vi "VALEW_ATC_Verify Concurrent All Valves.vi"(0 "GEA2 Reference In":refnum<k24>, 11 "Error In":errorcluster) -> (4 "GEA2 Reference Out":refnum<k24>, 6 "Pass/fail?":bool, 8 "Report Text":string, 15 "Error Out":errorcluster)   [LabVIEW 2016, in "TL27.lvlib"]
doc: "This test covers the ATC algorithm when doing a concurrent fill with ALL valves. A concurrent fill allows both hot and cold valves to be on at the same time. The valves are operated in parallel. When the cold valve is requested to be on, the fabric softener and spray valves also come on in this test."
uses:
  Projects/TL27.lvlib
  C:/Automation/DLLs/PC Dot Net/GeaCommunication.dll
  Common/LabVIEW GEA2 Toolkit/LabVIEW_GEA2_Toolkit.lvlibp/type defs/Source_Destination.ctl
  Valew Common/type defs/MC_Cycle_Engine_Request_State.ctl
  Common/LabVIEW GEA2 Toolkit/LabVIEW_GEA2_Toolkit.lvlibp/type defs/ERD Write Data In.ctl
  Common/LabVIEW GEA2 Toolkit/LabVIEW_GEA2_Toolkit.lvlibp/type defs/Data Type.ctl
  Common/LabVIEW GEA2 Toolkit/LabVIEW_GEA2_Toolkit.lvlibp/type defs/ERD Read Data In.ctl
  <vilib>/DAQmx/write.llb/DAQmx Write (Analog DBL 1Chan 1Samp).vi
  <vilib>/DAQmx/create/channels.llb/DAQmx Create Channel (AO-Voltage-Basic).vi
  <vilib>/DAQmx/miscellaneous.llb/DAQmx Fill In Error Info.vi
  Common/LabVIEW GEA2 Toolkit/LabVIEW_GEA2_Toolkit.lvlibp
panel:
  out "Calc bath temp after seg gals":dbl
  out "Bath temp after seg gals":dbl
  out "Hot valve time (s) ATC":u16
  out "Cold valve time (s) ATC":u16
  out "Bath temp updated after segment fill?":bool
  out "Valve ON Times (s)":dbl[](array[numeric])
  out "Cold valve pass?":bool
  out "Hot valve pass?":bool
  out "Cold valve time (s) Calc":dbl
  out "Hot valve time (s) Calc":dbl
  in  "Standalone?":bool
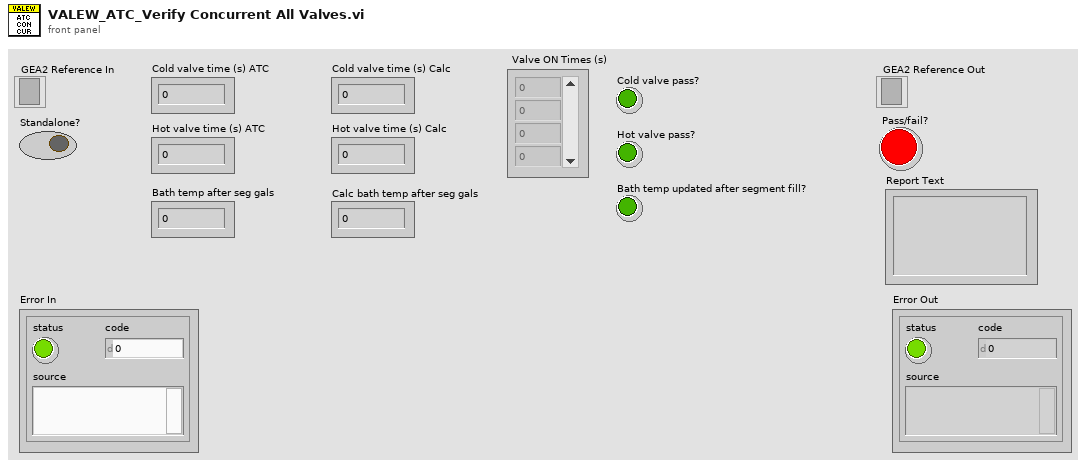
[diagram p1: front panel]
types:
  T1 = typedef "LabVIEW_GEA2_Toolkit.lvlibp/ERD Write Data In.ctl" = cluster{"ERD Number":u16, "Data Type":T2, "Data":string}
  T2 = typedef "LabVIEW_GEA2_Toolkit.lvlibp/Data Type.ctl" = enum16{"string", "boolean", "uint8_t", "uint16_t", "uint32_t", "uint64_t", "int8_t", "int16_t", "int32_t", "int64_t"}
  T3 = typedef "TL27.lvlib/MC_Cycle_Engine_Request_State.ctl" = enum16{"Select", "Start", "Pause", "Resume", "Stop"}
  T4 = typedef "LabVIEW_GEA2_Toolkit.lvlibp/ERD Read Data In.ctl" = cluster{"ERD Number":u16, "Data Type":T2}
  T5 = enum16{"EQ (==)", "NE (!=)", "GT (>)", "LT (<)", "GE (>=)", "LE (<=)", "GTLT(> <)", "GELE (>= <=)", "GELT (>= <)", "GTLE (> <=)", "LTGT (< >)", "LEGE (<= >=)", "LEGT (<= >)", "LTGE (< >=)", "No Comparison"}
  T6 = typedef "LabVIEW_GEA2_Toolkit.lvlibp/Source_Destination.ctl" = cluster{"Source":u8, "Destination":u8}
  T7 = typedef "TL27.lvlib/VALEW_ATC_Data.ctl" = cluster{"Accumulated hot gallons":dbl, "Accumulated cold gallons":dbl, "Current tub gallons":dbl, "Cold inlet temp (F)":dbl, "Hot inlet temp (F)":dbl, "Warm inlet temp (F)":dbl, "Hot valve time (s)":u16, "Cold valve time (s)":u16, "Current bath temp (F)":dbl, "Current water temp (F)":dbl, "Segment gallons":dbl}
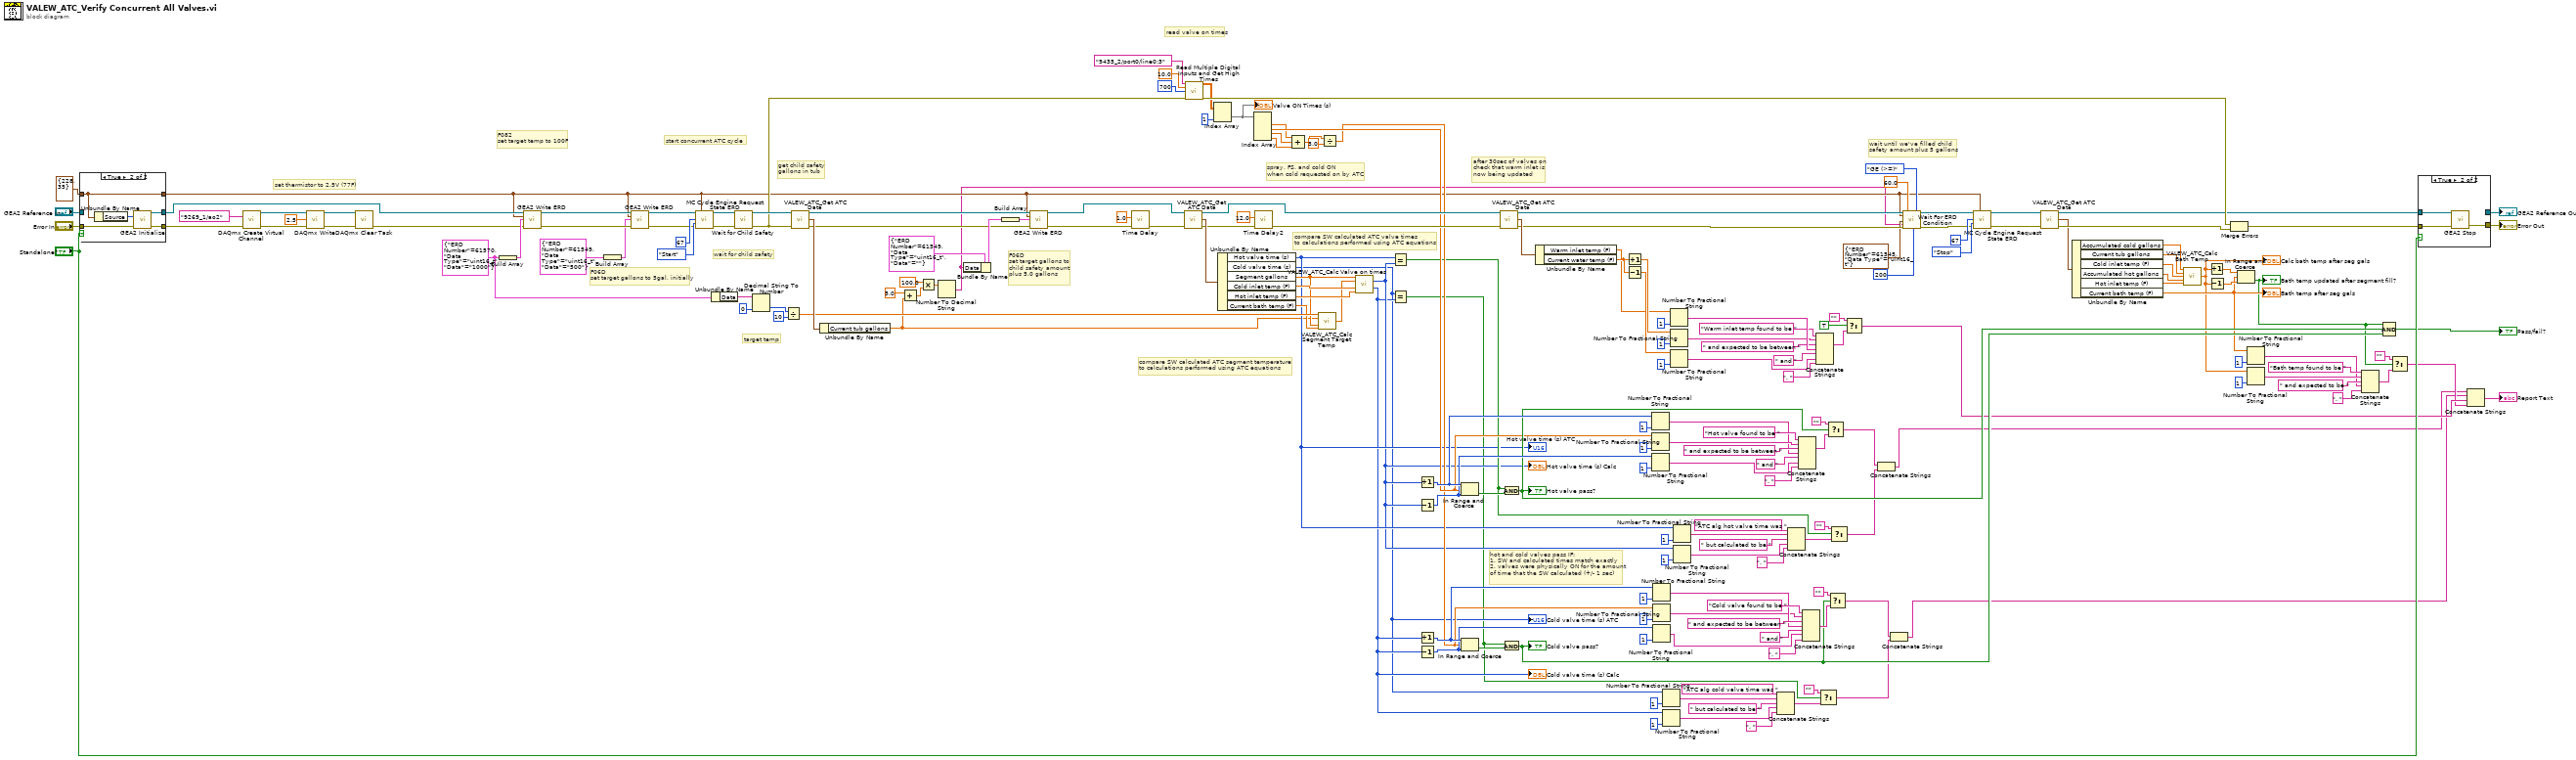
[diagram p0: block diagram]
diagram:
  w184 = T1 {"ERD Number"=61570, "Data Type"=enum."uint16_t", "Data"="1000"} ("ERD Write Data In")
  # "hot and cold valves pass IF:\n1. SW and calculated times match exactly\n2. valves were physically ON for the amount\nof time that the SW calculated (+/- 1 sec)"
  # "compare SW calculated ATC segment temperature\nto calculations performed using ATC equations"
  # "compare SW calculated ATC valve times\nto calculations performed using ATC equations"
  # "F06D\nset target gallons to\nchild safety amount\nplus 5.0 gallons"
  # "spray, FS, and cold ON\nwhen cold requested on by ATC"
  # "F06D\nset target gallons to 5gal, initially"
  # "after 30sec of valves on\ncheck that warm inlet is\nnow being updated"
  # "get child safety\ngallons in tub"
  # "wait until we've filled child \nsafety amount plus 5 gallons"
  # "read valve on times"
  # "target temp"
  # "set thermistor to 2.5V (77F)"
  # "wait for child safety"
  # "start concurrent ATC cycle"
  # "F082\nset target temp to 100F"
  n1 = case shown="True" "Standalone?" {
    tunnel: T6 {"Source"=228, "Destination"=35} ("GEA Inputs") -> [w195 w198]
    tunnel: [w197 w201] -> w48
    tunnel: [w196 w200] -> w138
    tunnel: "Error In" -> [w196 w199]
    tunnel: "GEA2 Reference In" -> [w197 _]
    tunnel: [w195 w198] -> w5
    frame False {
    }
    frame True {
      n2 = Unbundle By Name(w198) -> ("Source"=w202:u8)
      n3 = call "GEA2 Initialize.vi"("Source Address"=w202, "error in"=w199) -> ("GEA2 Reference Out"=w201:refnum<k24>, "error out"=w200:errorcluster)  [unwired: 11 in, 1 out]
    }
  }
  n4 = call-poly <vilib>:"DAQmx Create Virtual Channel.vi"("physical channels"=tag "9269_1/ao2", "error in"=w138) -> ("task out"=w170:refnum<k21>, "error out"=w169:errorcluster)  [unwired: 12 in]
  n5 = call-poly <vilib>:"DAQmx Write.vi"("task/channels in"=w170, "data"=2.5, "error in"=w169) -> ("task out"=w136:refnum<k21>, "error out"=w137:errorcluster)  [unwired: 10 in, 1 out]
  n6 = call <vilib>:"DAQmx Clear Task.vi"("task in"=w136, "error in"=w137) -> ("error out"=w49:errorcluster)  [unwired: 13 in]
  n7 = Build Array(w184) -> (w183:T1[])
  n8 = call "GEA2 Write ERD.vi"("GEA2 Reference In"=w48, "GEA Inputs"=w5, "Write ERD List"=w183, "Error In"=w49) -> ("GEA2 Reference Out"=w165:refnum<k24>, "Error Out"=w164:errorcluster)  [unwired: 9 in, 1 out]
  n9 = Build Array(T1 {"ERD Number"=61549, "Data Type"=enum."uint16_t", "Data"="500"} ("ERD Write Data In")) -> (w131:T1[])
  n10 = call "GEA2 Write ERD.vi"("GEA2 Reference In"=w165, "GEA Inputs"=w5, "Write ERD List"=w131, "Error In"=w164) -> ("GEA2 Reference Out"=w162:refnum<k24>, "Error Out"=w163:errorcluster)  [unwired: 9 in, 1 out]
  n11 = call "MC Cycle Engine Request State ERD.vi"("GEA2 Reference In"=w162, "GEA Inputs"=w5, "Cycle #"=u8 67, "MC Cycle Engine State"=MC_Cycle_Engine_Request_State."Start", "Error In"=w163) -> ("GEA2 Reference Out"=w189:refnum<k24>, "Error Out"=w161:errorcluster)  [unwired: 9 in]
  n12 = Unbundle By Name(w184) -> ("Data"=w182:string)
  n13 = call "Wait for Child Safety.vi"("GEA2 Reference In"=w189, "Error In"=w161) -> ("GEA2 Reference Out"=w160:refnum<k24>, "Error Out"=w47:errorcluster)  [unwired: 9 in, 3 out]
  n14 = Decimal String To Number(string=w182, default (0L)=u16 0 ("default (0 U32)")) -> (number=w180:u16)  [unwired: 1 in, 1 out]
  n15 = Divide(x=w180, y=u16 10) -> (x/y=w134:dbl)
  n16 = call "VALEW_ATC_Get ATC Data.vi"("GEA2 Reference In"=w160, "Error In"=w47) -> ("GEA2 Reference Out"=w9:refnum<k24>, "ATC Data"=w159:T7, "Error Out"=w8:errorcluster)  [unwired: 11 in]
  n17 = Unbundle By Name(w159) -> ("Current tub gallons"=w4:dbl)
  n18 = Add(x=5.0, y=w4) -> (x+y=w11:dbl)
  n19 = Multiply(x=100.0, y=w11) -> (x*y=w12:dbl)
  n20 = Number To Decimal String(number=w12) -> (decimal integer string=w3:string)  [unwired: 1 in]
  n21 = Bundle By Name(cluster=T1 {"ERD Number"=61549, "Data Type"=enum."uint16_t", "Data"=""} ("ERD Write Data In"), "Data"=w3) -> (w13:T1)
  n22 = Build Array(w13) -> (w16:T1[])
  n23 = call "GEA2 Write ERD.vi"("GEA2 Reference In"=w9, "GEA Inputs"=w5, "Write ERD List"=w16, "Error In"=w8) -> ("GEA2 Reference Out"=w7:refnum<k24>, "Error Out"=w6:errorcluster)  [unwired: 9 in, 1 out]
  n24 = call "Time Delay"("error in (no error)"=w6, "Delay Time (s)"=1.0) -> ("error out"=w187:errorcluster)  [unwired: 9 in]
  n25 = call "VALEW_ATC_Get ATC Data.vi"("GEA2 Reference In"=w7, "Error In"=w187) -> ("GEA2 Reference Out"=w172:refnum<k24>, "ATC Data"=w186:T7, "Error Out"=w174:errorcluster)  [unwired: 11 in]
  n26 = call "Read Multiple Digital Inputs and Get High Times.vi"("Lines"=tag "9435_2/port0/line0:3", "Rate (Hz)"=10.0 ("rate"), "Samples"=700 ("samples per channel"), "Error In"=w47) -> ("High Times (s)"=w149:dbl[][], "Error Out"=w166:errorcluster)  [unwired: 10 in]
  n27 = Index Array(array=w149, index (col)=1 ("disabled index (col)")) -> (element=w63:dbl[])  [unwired: 1 in]
  "Valve ON Times (s)" <- w63
  n28 = Unbundle By Name(w186) -> ("Hot valve time (s)"=w33:u16, "Cold valve time (s)"=w21:u16, "Segment gallons"=w133:dbl, "Cold inlet temp (F)"=w150:dbl, "Hot inlet temp (F)"=w185:dbl, "Current bath temp (F)"=w132:dbl)
  "Cold valve time (s) ATC" <- w21
  "Hot valve time (s) ATC" <- w33
  n29 = Index Array(array=w63) -> (element #1=w57:dbl, element #2=w62:dbl, element #3=w61:dbl, element #4=w60:dbl)  [unwired: 4 in]
  n30 = call "Time Delay2"("error in (no error)"=w174, "Delay Time (s)"=12.0) -> ("error out"=w173:errorcluster)  [unwired: 9 in]
  n31 = Compound Arithmetic op=ADD(w57, w61, w60) -> (w59:dbl)
  n32 = call "VALEW_ATC_Calc Segment Target Temp.vi"("T(target)"=w134, "V(bath)"=w4, "V(segment)"=w133, "T(bath)"=w132) -> ("T(segment target)"=w135:dbl)  [unwired: 11 in]
  n33 = Divide(x=w59, y=3.0) -> (x/y=w56:dbl)
  n34 = call "VALEW_ATC_Calc Valve on times.vi"("V(segment)"=w133, "T(segment target)"=w135, "T(cold inlet)"=w150, "T(hot inlet)"=w185) -> ("t(hot valve)"=w32:u16, "t(cold valve)"=w22:u16)  [unwired: 10 in]
  "Hot valve time (s) Calc" <- w32
  "Cold valve time (s) Calc" <- w22
  n35 = Equal?(x=w33, y=w32) -> (x = y?=w34:bool)
  n36 = Equal?(x=w21, y=w22) -> (x = y?=w20:bool)
  n37 = Increment(x=w32) -> (x+1=w125:u16)
  n38 = Decrement(x=w32) -> (x-1=w120:u16)
  n39 = Increment(x=w22) -> (x+1=w118:u16)
  n40 = Decrement(x=w22) -> (x-1=w117:u16)
  n41 = In Range and Coerce(upper limit=w125, x=w62, lower limit=w120) -> (In Range?=w148:bool)  [unwired: 1 out]
  n42 = In Range and Coerce(upper limit=w118, x=w56, lower limit=w117) -> (In Range?=w147:bool)  [unwired: 1 out]
  n43 = call "VALEW_ATC_Get ATC Data.vi"("GEA2 Reference In"=w172, "Error In"=w173) -> ("GEA2 Reference Out"=w157:refnum<k24>, "ATC Data"=w171:T7, "Error Out"=w158:errorcluster)  [unwired: 11 in]
  n44 = And(x=w34, y=w148) -> (x .and. y?=w100:bool)
  "Hot valve pass?" <- w100
  n45 = And(x=w20, y=w147) -> (x .and. y?=w99:bool)
  "Cold valve pass?" <- w99
  n46 = Unbundle By Name(w171) -> ("Warm inlet temp (F)"=w2:dbl, "Current water temp (F)"=w146:dbl)
  n47 = Increment(x=w146) -> (x+1=w85:dbl)
  n48 = Decrement(x=w146) -> (x-1=w84:dbl)
  n49 = Number To Fractional String(number=w125, precision (6)=i16 1) -> (F-format string=w113:string)  [unwired: 2 in]
  n50 = Number To Fractional String(number=w62, precision (6)=i16 1) -> (F-format string=w115:string)  [unwired: 2 in]
  n51 = Number To Fractional String(number=w120, precision (6)=i16 1) -> (F-format string=w111:string)  [unwired: 2 in]
  n52 = Number To Fractional String(number=w118, precision (6)=i16 1) -> (F-format string=w104:string)  [unwired: 2 in]
  n53 = Number To Fractional String(number=w56, precision (6)=i16 1) -> (F-format string=w103:string)  [unwired: 2 in]
  n54 = Number To Fractional String(number=w117, precision (6)=i16 1) -> (F-format string=w102:string)  [unwired: 2 in]
  n55 = Number To Fractional String(number=w21, precision (6)=i16 1) -> (F-format string=w26:string)  [unwired: 2 in]
  n56 = Number To Fractional String(number=w22, precision (6)=i16 1) -> (F-format string=w28:string)  [unwired: 2 in]
  n57 = Number To Fractional String(number=w2, precision (6)=i16 1) -> (F-format string=w93:string)  [unwired: 2 in]
  n58 = Number To Fractional String(number=w85, precision (6)=i16 1) -> (F-format string=w91:string)  [unwired: 2 in]
  n59 = Number To Fractional String(number=w84, precision (6)=i16 1) -> (F-format string=w95:string)  [unwired: 2 in]
  n60 = Number To Fractional String(number=w33, precision (6)=i16 1) -> (F-format string=w44:string)  [unwired: 2 in]
  n61 = Number To Fractional String(number=w32, precision (6)=i16 1) -> (F-format string=w42:string)  [unwired: 2 in]
  n62 = Concatenate Strings("ATC alg cold valve time was ", w26, " but calculated to be ", w28, ". " ("string")) -> (w31:string)
  n63 = Concatenate Strings("ATC alg hot valve time was ", w44, " but calculated to be ", w42, ". " ("string")) -> (w39:string)
  n64 = Concatenate Strings("Hot valve found to be ", w115, " and expected to be between ", w113, " and " ("string"), w111, ". " ("string")) -> (w109:string)
  n65 = Concatenate Strings("Cold valve found to be ", w103, " and expected to be between ", w104, " and " ("string"), w102, ". " ("string")) -> (w101:string)
  n66 = Concatenate Strings("Warm inlet temp found to be ", w91, " and expected to be between ", w93, " and " ("string"), w95, ". " ("string")) -> (w97:string)
  n67 = Select(t="", s=w20, f=w31) -> (s? t:f=w19:string)
  n68 = Select(t="", s=w100, f=w109) -> (s? t:f=w36:string)
  n69 = Select(t="", s=w99, f=w101) -> (s? t:f=w18:string)
  n70 = Select(t="", s=w34, f=w39) -> (s? t:f=w37:string)
  n71 = Select(t="", s=TRUE, f=w97) -> (s? t:f=w71:string)
  n72 = Concatenate Strings(w36, w37) -> (w35:string)
  n73 = Concatenate Strings(w18, w19) -> (w17:string)
  n74 = call "Wait For ERD Condition.vi"("GEA2 Reference In"=w157, "GEA Inputs"=w5, "ERD Read Data"=T4 {"ERD Number"=61545, "Data Type"=enum."uint16_t"}, "Expected Low"=w3, "Error In"=w158, "Timeout (s)"=60.0, "Loop Rate (ms)"=u32 200, "Comparison"=T5."GE (>=)") -> ("GEA2 Reference Out"=w55:refnum<k24>, "Error Out"=w52:errorcluster)  [unwired: 7 in, 3 out]
  n75 = call "MC Cycle Engine Request State ERD.vi"("GEA2 Reference In"=w55, "GEA Inputs"=w5, "Cycle #"=u8 67, "MC Cycle Engine State"=MC_Cycle_Engine_Request_State."Stop", "Error In"=w52) -> ("GEA2 Reference Out"=w54:refnum<k24>, "Error Out"=w53:errorcluster)  [unwired: 9 in]
  n76 = call "VALEW_ATC_Get ATC Data.vi"("GEA2 Reference In"=w54, "Error In"=w53) -> ("GEA2 Reference Out"=w51:refnum<k24>, "ATC Data"=w151:T7, "Error Out"=w152:errorcluster)  [unwired: 11 in]
  n77 = Unbundle By Name(w151) -> ("Accumulated cold gallons"=w141:dbl, "Current tub gallons"=w142:dbl, "Cold inlet temp (F)"=w143:dbl, "Accumulated hot gallons"=w144:dbl, "Hot inlet temp (F)"=w145:dbl, "Current bath temp (F)"=w75:dbl)
  "Bath temp after seg gals" <- w75
  n78 = call "VALEW_ATC_Calc Bath Temp.vi"("V(bath cold)"=w141, "V(bath)"=w142, "T(cold inlet)"=w143, "V(bath hot)"=w144, "T(hot inlet)"=w145) -> ("T(bath)"=w74:dbl)  [unwired: 10 in]
  "Calc bath temp after seg gals" <- w74
  n79 = Increment(x=w74) -> (x+1=w139:dbl)
  n80 = Decrement(x=w74) -> (x-1=w140:dbl)
  n81 = Merge Errors(w166, w152) -> (w50:errorcluster)
  n82 = In Range and Coerce(upper limit=w139, x=w75, lower limit=w140) -> (In Range?=w72:bool)  [unwired: 1 out]
  "Bath temp updated after segment fill?" <- w72
  n83 = Number To Fractional String(number=w75, precision (6)=i16 1) -> (F-format string=w77:string)  [unwired: 2 in]
  n84 = Number To Fractional String(number=w74, precision (6)=i16 1) -> (F-format string=w79:string)  [unwired: 2 in]
  n85 = Concatenate Strings("Bath temp found to be ", w79, " and expected to be ", w77, ". " ("string")) -> (w76:string)
  n86 = Compound Arithmetic op=AND(w72, w100, w99) -> (→"Pass/fail?":bool)
  n87 = Select(t="", s=w72, f=w76) -> (s? t:f=w70:string)
  n88 = case shown="True" "Standalone?" {
    tunnel: w50 -> [w204 w207]
    tunnel: w51 -> [w203 w206]
    tunnel: [w204 w205] -> w68
    tunnel: [w203 _] -> w129
    frame False {
    }
    frame True {
      n89 = call "GEA2 Stop.vi"("GEA2 Reference In"=w206, "Error In"=w207) -> ("Error Out"=w205:errorcluster)  [unwired: 13 in]
    }
  }
  "GEA2 Reference Out" <- w129
  "Error Out" <- w68
  n90 = Concatenate Strings(w35, w17, w71, w70) -> (→"Report Text":string)
